vi "oa_(SubVI).vi"(9 "XYZ":dbl[](array[numeric]) format="%0.2f", 10 "a":dbl[](array[numeric]) format="%0.2f", 11 "o":dbl[](array[numeric]) format="%0.2f") -> (0 "POSE":dbl[](array[numeric]), 1 "RPY":cluster{"roll":dbl, "pitch":dbl, "yaw":dbl}, 2 "euler ZYZ":T1, 3 "Array":dbl[][](array[numeric]))   [LabVIEW 2015]
uses:
  <vilib>/Analysis/baseanly.llb/Unit Vector (DBL).vi
  <vilib>/Analysis/coordinate.llb/Direction Cosines To Euler Angles.vi
  <vilib>/Analysis/NI_AALBase.lvlib
  <vilib>/Analysis/NI_AALPro.lvlib
  <vilib>/robotics/Kinematics/NI_Kinematics.lvlib
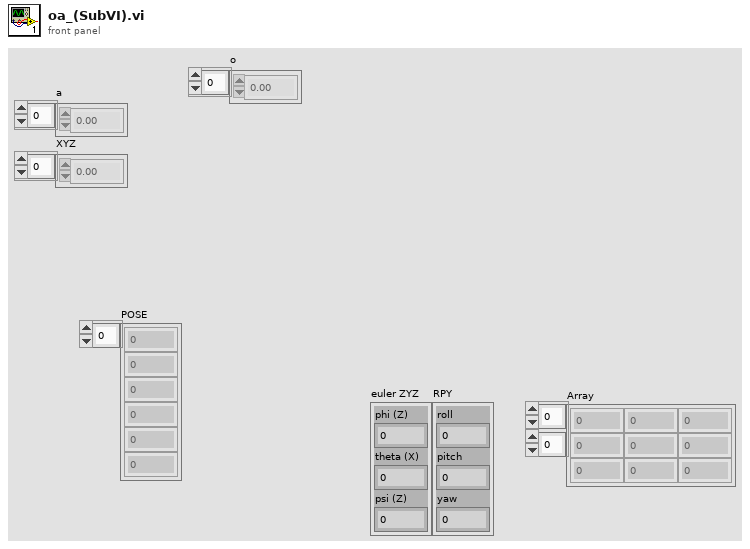
[diagram p1: front panel]
types:
  T1 = cluster{"phi (Z)":dbl, "theta (X)":dbl, "psi (Z)":dbl}
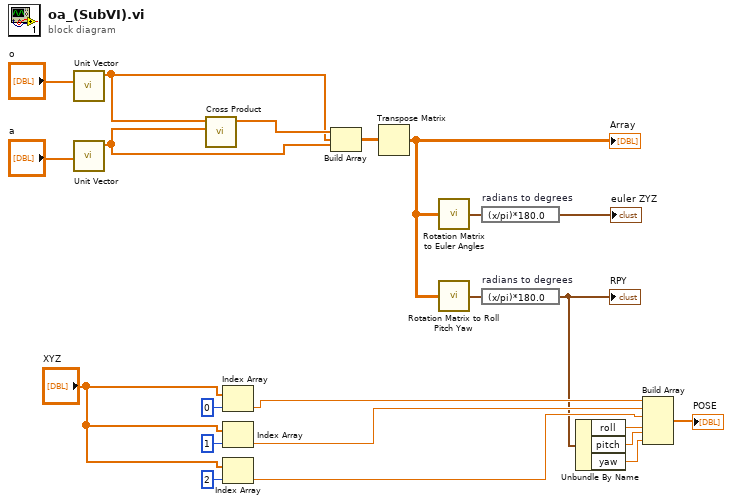
[diagram p0: block diagram]
diagram:
  n1 = call-poly <vilib>:"Unit Vector.vi"("Input Vector"="o") -> ("Unit Vector"=w19:dbl[])  [unwired: 8 in, 2 out]
  n2 = call-poly <vilib>:"Unit Vector.vi"("Input Vector"="a") -> ("Unit Vector"=w18:dbl[])  [unwired: 8 in, 2 out]
  n3 = call <vilib>:"Cross Product.vi"("B Vector"=w18, "A Vector"=w19) -> ("Cross Product"=w20:dbl[])  [unwired: 8 in, 1 out]
  n4 = Index Array(array="XYZ", index=0) -> (element=w10:dbl)
  n5 = Index Array(array="XYZ", index=1) -> (element=w9:dbl)
  n6 = Index Array(array="XYZ", index=2) -> (element=w8:dbl)
  n7 = Build Array(w20, w19, w18) -> (w15:dbl[][])
  n8 = Transpose Matrix(1:w15) -> (0:w1:dbl[][])
  "Array" <- w1
  n9 = call <vilib>:"Rotation Matrix to Euler Angles.vi"("rotation matrix"=w1) -> ("euler angles"=w17:T1)
  n10 = call <vilib>:"Rotation Matrix to Roll Pitch Yaw.vi"("rotation matrix"=w1) -> ("angles"=w14:cluster{"roll":dbl, "pitch":dbl, "yaw":dbl})
  n11 = expression code="(x/pi)*180.0" "radians to degrees"(w17) -> (→"euler ZYZ":T1)
  n12 = expression code="(x/pi)*180.0" "radians to degrees"(w14) -> (w2:cluster{"roll":dbl, "pitch":dbl, "yaw":dbl})
  "RPY" <- w2
  n13 = Unbundle By Name(w2) -> ("roll"=w11:dbl, "pitch"=w12:dbl, "yaw"=w13:dbl)
  n14 = Build Array(w10, w9, w8, w11, w12, w13) -> (→"POSE":dbl[])
